vi "Autonomous Independent.vi"() -> ()   [LabVIEW 2016]
doc: "This VI is called when autonomous begins, and will automatically be terminated when autonomous ends. You can carry out timed or sensor driven robot movement independently without needing to return to the caller."
uses:
  <vilib>/Rock Robotics/WPI/Utilities/WPI_GetSetVariantRefNum.vi
  Robot Global Data.vi
  <vilib>/addons/control/pid/pid.llb/PID (DBL).vi
  Libraries/navX Library v2/navX Library v2.lvlib
  <vilib>/addons/control/pid/NI_PID_pid.lvlib
panel:
  out "32bit integer":i32
  # "Be sure to right-click and choose Data Operations>>Make Current Value default if you want to save the array values with the VI"
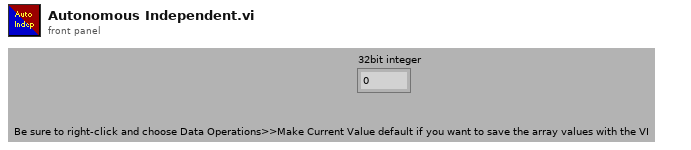
[diagram p1: front panel]
types:
  T1 = typedef "WPI_AnalogChannelDevRef.ctl" = cluster{"DevStatus":errorcluster, "Analog Channel":T2}
  T2 = typedef "FPGA_AIChannel.ctl" = enum8{"AI 0", "AI 1", "AI 2", "AI 3", "AI MXP 0", "AI MXP 1", "AI MXP 2", "AI MXP 3", "Invalid"}
  T3 = typedef "navX Library v2.lvlib/Z900_navX_DeviceTypeDef.ctl" = cluster{"Interface":cluster{"Protocol":T4, "Update Rate (4Hz-100Hz)":u8, "navX Open TypeDef":variant}, "Notify Packet":refnum<notifier>, "Loop VI Refnum":refnum<vi>, "Ready to Close Occurrence Refnum":refnum<k4>}
  T4 = typedef "navX Library v2.lvlib/Z900_navX_ProtocolTypeDef.ctl" = enum16{"SERIAL", "I2C", "SPI"}
  T5 = typedef "WPI_RobotDriveDevRef.ctl" = cluster{"DevStatus":errorcluster, "Motors[]":T6[], "Square Inputs":bool, "Max Output":dbl}
  T6 = typedef "WPI_MotorControlDeviceRef.ctl" = cluster{"DeviceStatus":errorcluster, "Type":T7, "PWM":cluster{"PWM Channel":T8, "DeadBand":T9}, "CAN":cluster{"Device Number":u8, "SetOutput VI Ref":variant, "GetOutput VI Ref":variant, "Enable VI Ref":variant, "Disable VI Ref":variant, "Data":variant}, "Invert":bool}
  T7 = typedef "WPI_MotorControlType.ctl" = enum16{"PWM", "CAN"}
  T8 = typedef "FPGA_DIOPWMChannel.ctl" = enum8{"PWM 0", "PWM 1", "PWM 2", "PWM 3", "PWM 4", "PWM 5", "PWM 6", "PWM 7", "PWM 8", "PWM 9", "PWM MXP 0", "PWM MXP 1", "PWM MXP 2", "PWM MXP 3", "PWM MXP 4", "PWM MXP 5", "PWM MXP 6", "PWM MXP 7", "PWM MXP 8", "PWM MXP 9", "Invalid"}
  T9 = typedef "WPI_PWMDeadband.ctl" = cluster{"Name":string, "maxPositivePwm":i32, "minPositivePwm":i32, "centerPwm":i32, "maxNegativePwm":i32, "minNegativePwm":i32, "angularRange":u16}
  T10 = typedef "WPI_DigitalInputDevRef.ctl" = cluster{"DevStatus":errorcluster, "DIO Channel":T11}
  T11 = typedef "FPGA_DIOChannel.ctl" = enum8{"DIO 0", "DIO 1", "DIO 2", "DIO 3", "DIO 4", "DIO 5", "DIO 6", "DIO 7", "DIO 8", "DIO 9", "DIO MXP 0", "DIO MXP 1", "DIO MXP 2", "DIO MXP 3", "DIO MXP 4", "DIO MXP 5", "DIO MXP 6", "DIO MXP 7", "DIO MXP 8", "DIO MXP 9", "DIO MXP 10", "DIO MXP 11", "DIO MXP 12", "DIO MXP 13", "DIO MXP 14", "DIO MXP 15", "SPI Port CS1", "SPI Port CS2", "SPI Port CS3", "SPI Port MISO", "SPI Port MOSI", "Invalid"}
  T12 = cluster{"proportional gain (Kc)":dbl, "integral time (Ti, min)":dbl, "derivative time (Td, min)":dbl}
  T13 = cluster{"Yaw":dbl, "Roll":dbl, "Pitch":dbl, "Heading":dbl, "Fused Heading":dbl}
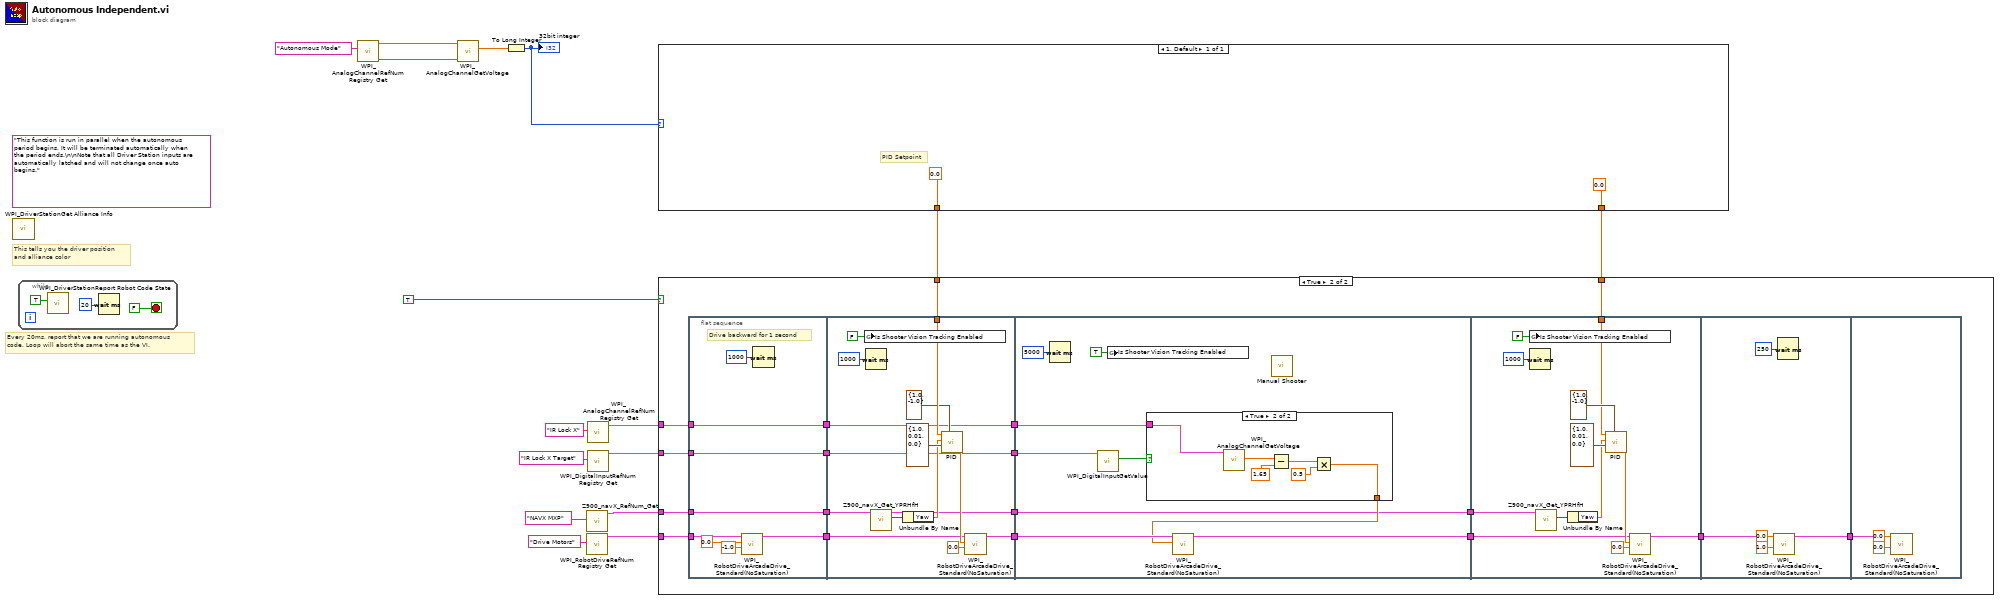
[diagram p0: block diagram]
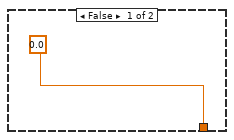
[diagram p3: hidden frame]
diagram:
  (unwired) "This function is run in parallel when the autonomous period begins. It will be terminated automatically when the period ends.\n\nNote that all Driver Station inputs are automatically latched and will not change once auto begins."
  # "Every 20ms, report that we are running autonomous\ncode. Loop will abort the same time as the VI."
  # "This tells you the driver position\nand alliance color"
  n1 = call <vilib>:"WPI_DriverStationGet Alliance Info.vi"() -> ()  [unwired: 12 out]
  n2 = while {
    stop <- FALSE stop-if-true
    n3 = call <vilib>:"WPI_DriverStationReport Robot Code State.vi"("Autonomous"=TRUE) -> ()  [unwired: 10 in, 1 out]
    n4 = Wait (ms)(milliseconds to wait=u32 20) -> ()  [unwired: 1 out]
  }
  n5 = call <vilib>:"WPI_AnalogChannelRefNum Registry Get.vi"("refnum name"="Autonomous Mode") -> ("error out"=w14:errorcluster, "AIDeviceRef"=w15:T1)  [unwired: 9 in]
  n6 = call <vilib>:"WPI_AnalogChannelGetVoltage.vi"("error in (no error)"=w14, "AIDeviceRef"=w15) -> ("Voltage"=w13:dbl)  [unwired: 7 in, 2 out]
  n7 = To Long Integer(number=w13) -> (32bit integer=w12:i32)
  "32bit integer" <- w12
  n8 = call "Z900_navX_RefNum_Get.vi"("refnum name"="NAVX MXP") -> ("navX Device"=w7:T3)  [unwired: 9 in, 1 out]
  n9 = call <vilib>:"WPI_RobotDriveRefNum Registry Get.vi"("refnum name"="Drive Motors") -> ("RobotDriveDevRef"=w9:T5)  [unwired: 1 in, 9 out]
  n10 = call <vilib>:"WPI_AnalogChannelRefNum Registry Get.vi"("refnum name"="IR Lock X") -> ("AIDeviceRef"=w2:T1)  [unwired: 9 in, 1 out]
  n11 = call <vilib>:"WPI_DigitalInputRefNum Registry Get.vi"("refnum name"="IR Lock X Target") -> ("DigitalInputDevRef"=w4:T10)  [unwired: 9 in, 1 out]
  n12 = case shown="1, Default" w12 {
    tunnel: [0.0 ("setpoint")] -> w6
    tunnel: [0.0 ("setpoint")] -> w1
    frame 1, Default {
      # "PID Setpoint"
    }
  }
  n13 = case shown="True" TRUE {
    tunnel: w9 -> [_ w39]
    tunnel: w7 -> [_ w36]
    tunnel: w6 -> [_ w35]
    tunnel: w4 -> [_ w32]
    tunnel: w2 -> [_ w29]
    tunnel: w1 -> [_ w24]
    frame False {
    }
    frame True {
      n14 = flat-sequence {
        tunnel: w39 -> [w47]
        tunnel: [w44] -> w38
        tunnel: [w43] -> w37
        tunnel: w36 -> [w43]
        tunnel: [w41] -> w33
        tunnel: w32 -> [w41]
        tunnel: [w40] -> w30
        tunnel: w29 -> [w40]
        tunnel: w38 -> [w57]
        tunnel: w37 -> [w56]
        tunnel: w35 -> [w58]
        tunnel: [w52] -> w34
        tunnel: w33 -> [w52]
        tunnel: [w51] -> w31
        tunnel: w30 -> [w50]
        tunnel: [w50] -> w28
        tunnel: [w49] -> w25
        tunnel: w34 -> [w70]
        tunnel: w31 -> [w69]
        tunnel: w28 -> [w67]
        tunnel: [w64] -> w27
        tunnel: [w63] -> w26
        tunnel: w25 -> [w63]
        tunnel: w27 -> [w83]
        tunnel: w26 -> [w82]
        tunnel: w24 -> [w81]
        tunnel: [w79] -> w23
        tunnel: w23 -> [w92]
        tunnel: [w91] -> w22
        tunnel: w22 -> [w96]
        frame #0 {
          # "Drive backward for 1 second"
          n15 = call <vilib>:"WPI_RobotDriveArcadeDrive_Standard(NoSaturation).vi"("Y axis value"=-1.0, "X axis value"=0.0, "RobotDriveDevRef"=w47) -> ("RobotDriveDevRef"=w44:T5)  [unwired: 1 in, 7 out]
          n16 = Wait (ms)(milliseconds to wait=u32 1000) -> ()  [unwired: 1 out]
        }
        frame #1 {
          n17 = global write "Robot Global Data.vi" "Is Shooter Vision Tracking Enabled"(FALSE ("Is Shooter Vision Tracking Enabled")) -> ()
          n18 = Wait (ms)(milliseconds to wait=u32 1000) -> ()  [unwired: 1 out]
          n19 = call "Z900_navX_Get_YPRHfH.vi"("navX Device"=w56) -> ("YRPHfH"=w61:T13, "navX Device"=w49:T3)  [unwired: 7 in, 2 out]
          n20 = Unbundle By Name(w61) -> ("Yaw"=w60:dbl)
          n21 = call-poly <vilib>:"PID.vi"("output range"=cluster{"output high":dbl, "output low":dbl} {"output high"=1.0, "output low"=-1.0}, "PID gains"=T12 {"proportional gain (Kc)"=1.0, "integral time (Ti, min)"=0.01, "derivative time (Td, min)"=0.0}, "process variable"=w60, "setpoint"=w58) -> ("output"=w59:dbl)  [unwired: 6 in, 1 out]
          n22 = call <vilib>:"WPI_RobotDriveArcadeDrive_Standard(NoSaturation).vi"("Y axis value"=0.0, "X axis value"=w59, "RobotDriveDevRef"=w57) -> ("RobotDriveDevRef"=w51:T5)  [unwired: 1 in, 7 out]
        }
        frame #2 {
          n23 = Wait (ms)(milliseconds to wait=u32 5000) -> ()  [unwired: 1 out]
          n24 = call <vilib>:"WPI_DigitalInputGetValue.vi"("DigitalInputDevRef"=w70) -> ("Value"=w71:bool)  [unwired: 8 in, 2 out]
          n25 = global write "Robot Global Data.vi" "Is Shooter Vision Tracking Enabled"(TRUE ("Is Shooter Vision Tracking Enabled")) -> ()
          n26 = case shown="True" w71 {
            tunnel: [0.0 w74] -> w68
            tunnel: w67 -> [_ w73]
            frame False {
            }
            frame True {
              n27 = call <vilib>:"WPI_AnalogChannelGetVoltage.vi"("AIDeviceRef"=w73) -> ("Voltage"=w78:dbl)  [unwired: 8 in, 2 out]
              n28 = Subtract(x=w78, y=1.65) -> (x-y=w76:dbl)
              n29 = Multiply(x=w76, y=0.5) -> (x*y=w74:dbl)
            }
          }
          n30 = call <vilib>:"WPI_RobotDriveArcadeDrive_Standard(NoSaturation).vi"("X axis value"=w68, "RobotDriveDevRef"=w69) -> ("RobotDriveDevRef"=w64:T5)  [unwired: 2 in, 7 out]
          n31 = call "Manual Shooter.vi"() -> ()  [unwired: 12 in]
        }
        frame #3 {
          n32 = global write "Robot Global Data.vi" "Is Shooter Vision Tracking Enabled"(FALSE ("Is Shooter Vision Tracking Enabled")) -> ()
          n33 = Wait (ms)(milliseconds to wait=u32 1000) -> ()  [unwired: 1 out]
          n34 = call "Z900_navX_Get_YPRHfH.vi"("navX Device"=w82) -> ("YRPHfH"=w89:T13)  [unwired: 7 in, 3 out]
          n35 = Unbundle By Name(w89) -> ("Yaw"=w88:dbl)
          n36 = call-poly <vilib>:"PID.vi"("output range"=cluster{"output high":dbl, "output low":dbl} {"output high"=1.0, "output low"=-1.0}, "PID gains"=T12 {"proportional gain (Kc)"=1.0, "integral time (Ti, min)"=0.01, "derivative time (Td, min)"=0.0}, "process variable"=w88, "setpoint"=w81) -> ("output"=w87:dbl)  [unwired: 6 in, 1 out]
          n37 = call <vilib>:"WPI_RobotDriveArcadeDrive_Standard(NoSaturation).vi"("Y axis value"=0.0, "X axis value"=w87, "RobotDriveDevRef"=w83) -> ("RobotDriveDevRef"=w79:T5)  [unwired: 1 in, 7 out]
        }
        frame #4 {
          n38 = call <vilib>:"WPI_RobotDriveArcadeDrive_Standard(NoSaturation).vi"("Y axis value"=1.0, "X axis value"=0.0, "RobotDriveDevRef"=w92) -> ("RobotDriveDevRef"=w91:T5)  [unwired: 1 in, 7 out]
          n39 = Wait (ms)(milliseconds to wait=u32 250) -> ()  [unwired: 1 out]
        }
        frame #5 {
          n40 = call <vilib>:"WPI_RobotDriveArcadeDrive_Standard(NoSaturation).vi"("Y axis value"=0.0, "X axis value"=0.0, "RobotDriveDevRef"=w96) -> ()  [unwired: 1 in, 8 out]
        }
      }
    }
  }
